vi "Set Timeout.vi"(8 "error in (no error)":errorcluster, 10 "Timeout (s)":i32=3, 11 "Handle in":i32) -> (0 "error out":errorcluster, 3 "Handle out":i32)   [LabVIEW 2013, in "Thorlabs_MC2000B.lvlib"]
uses:
  <instrlib>/Thorlabs_MC2000B/Thorlabs_MC2000B.lvlib
  <instrlib>/Thorlabs_MC2000B/Library/MC2000CommandLibWin64.dll
  <instrlib>/Thorlabs_MC2000B/Library/MC2000CommandLibWin32.dll
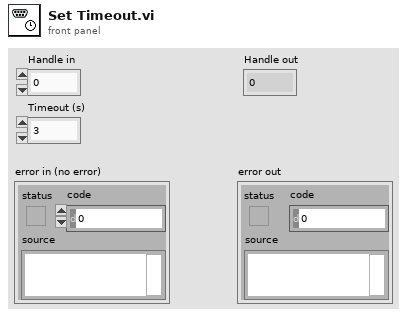
[diagram p1: front panel]
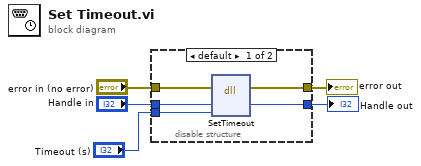
[diagram p0: block diagram]
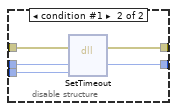
[diagram p2: hidden frame]
diagram:
  n1 = disable-structure shown="default" {
    disable-tunnel: "error in (no error)" -> [w10 w15]
    disable-tunnel: [w9 w14] -> w4
    disable-tunnel: "Timeout (s)" -> [w8 w13]
    disable-tunnel: "Handle in" -> [w7 w12]
    disable-tunnel: [w6 w11] -> w1
    frame condition #0 (active) {
      n2 = dll-call lib="C:/Program Files (x86)/National Instruments/LabVIEW 2013/instr.lib/Thorlabs_MC2000B/Library/MC2000CommandLibWin32.dll" fn="SetTimeout"(error in=w10, "Handle"=w7, "Timeout"=w8) -> (error out=w9:errorcluster, "Handle"=w6:i32)  [unwired: 4 in, 1 out]
    }
    frame condition #1 {
      n3 = dll-call lib="D:/Program Files/National Instruments/LabVIEW 2011/instr.lib/Thorlabs_MC2000B/Library/MC2000CommandLibWin64.dll" fn="SetTimeout"(error in=w15, "Handle"=w12, "Timeout"=w13) -> (error out=w14:errorcluster, "Handle"=w11:i32)  [unwired: 4 in, 1 out]
    }
  }
  "error out" <- w4
  "Handle out" <- w1
